vi "Actor Core.vi"(8 "error in":errorcluster, 11 "BuildServer in":refnum<class "BuildServer.lvclass">) -> (0 "error out":errorcluster, 3 "Actor out":refnum<class "Actor.lvclass">)   [LabVIEW 2017, in "BuildServer.lvlib" / "BuildServer.lvclass"]
doc: "(<B>Filename</B>: Actor Framework.lvlib:Actor.lvclass:Actor Core.vi)\n\nReceives messages to the actor, reacts to them, and initiates any error handling that may shut the actor down.\n\nDescendant classes may override this VI to append parallel tasks for the actor to complete while it handles messages. Overrides use the Call Parent Method node."
uses:
  BuildServer.lvclass
  <vilib>/ActorFramework/Actor/Actor.lvclass
  BuildServer Messages/Add LVProject Msg/Add LVProject Msg.lvclass
  BuildServer Messages/Update Project Organization Msg/Update Project Organization Msg.lvclass
  BuildServer Messages/Remove LVProject Msg/Remove LVProject Msg.lvclass
  BuildServer Messages/Add Tasks Msg/Add Tasks Msg.lvclass
  BuildServer Messages/Remove Tasks Msg/Remove Tasks Msg.lvclass
  BuildServer Messages/Sort TaskView Msg/Sort TaskView Msg.lvclass
  BuildServer Messages/Launch Task Settings Msg/Launch Task Settings Msg.lvclass
  <vilib>/ActorFramework/Stop Msg/Stop Msg.lvclass
  BuildServer Messages/Send Tasks To Workers Msg/Send Tasks To Workers Msg.lvclass
  BuildServer Messages/Start Tasks Msg/Start Tasks Msg.lvclass
  BuildServer Messages/Cancel Tasks Msg/Cancel Tasks Msg.lvclass
  BuildServer Messages/Stop Worker Msg/Stop Worker Msg.lvclass
  BuildServer Messages/Worker List Menu Selection Msg/Worker List Menu Selection Msg.lvclass
  <vilib>/Utility/sysdir.llb/System Directory Type.ctl
  BuildServer Messages/Task Update Message Msg/Task Update Message Msg.lvclass
  WebSocket Server/Actors/Actor wHelper/Actor wHelper/Actor wHelper.lvclass
  Volumes/Data/Users/benji667/Git/BuildFarm/WebSocket Server/Actors/Actor wHelper/Actor wHelper/Actor wHelper.lvclass
  Volumes/Data/Users/benji667/Git/BuildFarm/WebSocket Server/Actors/Actor wHelper/Actor wLauncher/Actor wLauncher.lvclass
  Volumes/Data/Users/benji667/Git/BuildFarm/WebSocket Server/Actors/Actor wHelper/Actor wUI/Actor wUI.lvclass
  Applications/National Instruments/LabVIEW 2017 64-bit/vi.lib/ActorFramework/Actor/Actor.lvclass
  ProjectOrganization.ctl
panel:
  in  "tasksSend":bool
  in  "projectsDelete":bool
  in  "tasksAdd":bool
  in  "projectsOpen":bool
  in  "tasksRemove":bool
  in  "workerKill":bool
  in  "taskSettings":bool
  in  "taskCancel":bool
  in  "taskStart":bool
  in  "projectOrganization":T1
  in  "ProjectsView":string[](tree)
  in  "TasksView":i32[](listbox)
  out "Status":string
  out "#proc":i32 caption="# of logical processors"
  out "WorkerList":string[][](array[string])
  # "LabVIEW Projects"
  # "Tasks"
  # "Status"
  # "Workers"
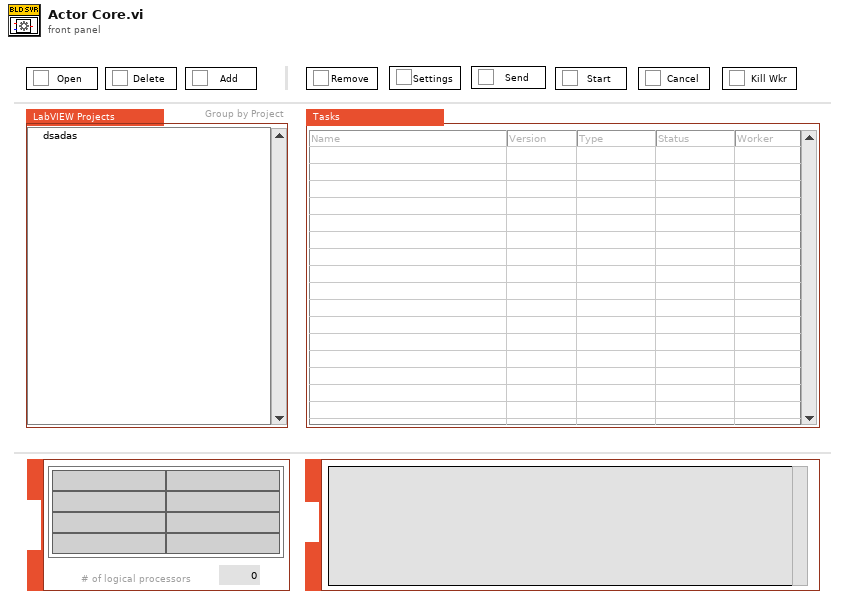
[diagram p1: front panel]
types:
  T1 = typedef "BuildServer.lvlib/BuildServer.lvclass/ProjectOrganization.ctl" = enum16{"Group by Project", "Group by Target", "Group by Type", "Group by Name"}
  T2 = cluster{"Properties:StopHelperLoop Reg Ref":refnum<event-registration>, "Properties:Msg Update Event":refnum<event-registration>, "Properties:New Worker Event":refnum<event-registration>}
  T3 = typedef "System Directory Type.ctl" = i32
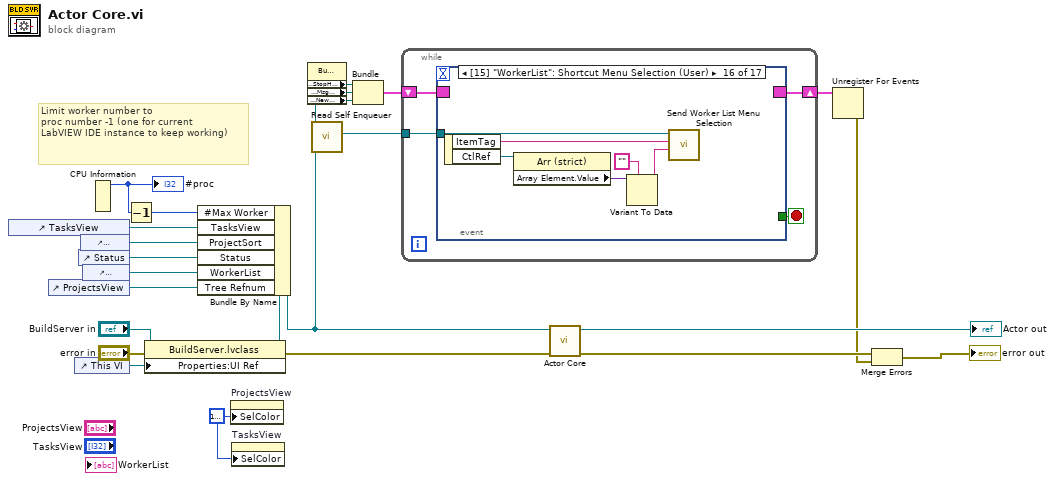
[diagram p0: block diagram]
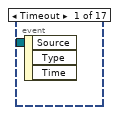
[diagram p2: hidden frame]
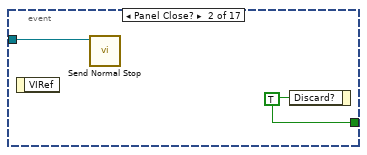
[diagram p3: hidden frame]
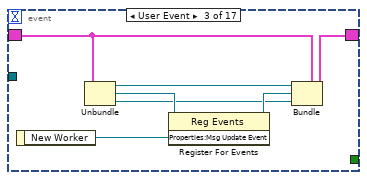
[diagram p4: hidden frame]
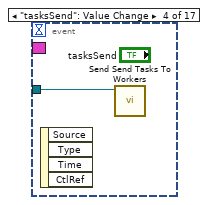
[diagram p5: hidden frame]
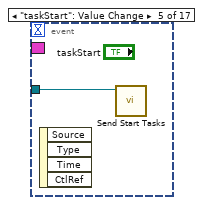
[diagram p6: hidden frame]
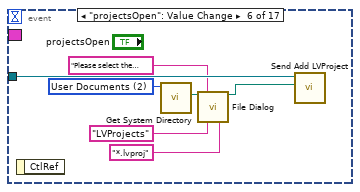
[diagram p7: hidden frame]
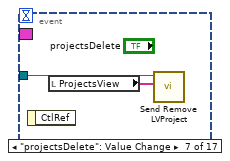
[diagram p8: hidden frame]
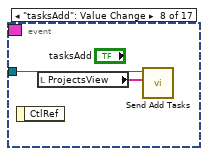
[diagram p9: hidden frame]
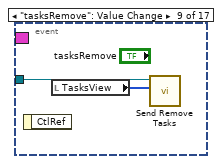
[diagram p10: hidden frame]
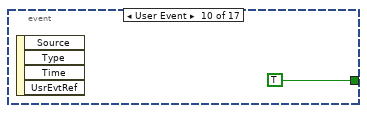
[diagram p11: hidden frame]
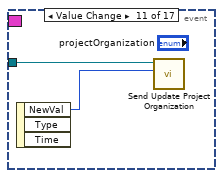
[diagram p12: hidden frame]
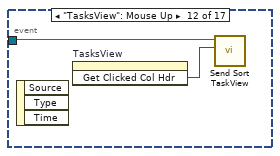
[diagram p13: hidden frame]
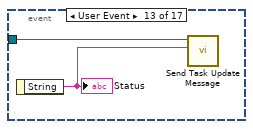
[diagram p14: hidden frame]
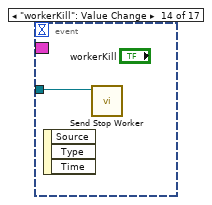
[diagram p15: hidden frame]
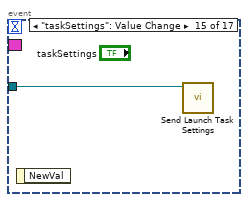
[diagram p16: hidden frame]
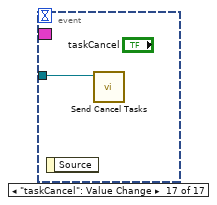
[diagram p17: hidden frame]
diagram:
  w13 = u32 16777224 ("Selection Color")
  # "Limit worker number to\nproc number -1 (one for current\nLabVIEW IDE instance to keep working)"
  n1 = control-ref of="TasksView"() -> (w14:refnum<vi>)
  n2 = control-ref of="ProjectsView"() -> (w19:refnum<vi>)
  n3 = control-ref of="This VI"() -> (w3:refnum<vi>)
  n4 = control-ref of="Status"() -> (w16:refnum<vi>)
  n5 = control-ref of="projectOrganization"() -> (w15:refnum<vi>)
  n6 = control-ref of="WorkerList"() -> (w17:refnum<vi>)
  n7 = CPU Information() -> (4:w10:i32)  [unwired: 3 out]
  "#proc" <- w10
  n8 = Decrement(x=w10) -> (x-1=w9:i32)
  n9 = property class="BuildServer.lvclass"(reference="BuildServer in", error in="error in", "Properties:UI Ref"=w3) -> (reference out=w5:refnum<class "BuildServer.lvclass">, error out=w1:errorcluster)
  n10 = Bundle By Name(cluster=w5, "#Max Worker"=w9, "TasksView"=w14, "ProjectSort"=w15, "Status"=w16, "WorkerList"=w17, "Tree Refnum"=w19) -> (w2:refnum<class "BuildServer.lvclass">)
  n11 = property on="ProjectsView" class="Tree (strict)"("SelColor"=w13) -> ()  [unwired: 2 in, 2 out]
  n12 = property on="TasksView" class="MCListbox (strict)"("SelColor"=w13) -> ()  [unwired: 2 in, 2 out]
  n13 = property class="BuildServer.lvclass"(reference=w2) -> ("Properties:StopHelperLoop Reg Ref"=w21:refnum<event-registration>, "Properties:Msg Update Event"=w8:refnum<event-registration>, "Properties:New Worker Event"=w6:refnum<event-registration>)  [unwired: 1 in, 2 out]
  n14 = call <vilib>:"Read Self Enqueuer.vi"("Actor"=w2) -> ("Self Enqueuer"=w18:refnum<class "Message Enqueuer.lvclass">)  [unwired: 10 in]
  n15 = Bundle("Properties:StopHelperLoop Reg Ref"=w21, "Properties:Msg Update Event"=w8, "Properties:New Worker Event"=w6) -> (w20:T2)  [unwired: 1 in]
  n16 = while {
    tunnel: w18 -> [w26]
    shift-right: [w25] -> w7
    shift-left: w20 -> [w27]
    stop <- w28 stop-if-true
    n17 = event shown="[15] \"WorkerList\": Shortcut Menu Selection (User)" {
      selector: w27 -> [_ _ w37 _ _ _ _ _ _ _ _ _ _ _ _ _ _]
      dyn-events: [_ _ w35 _ _ _ _ _ _ _ _ _ _ _ _ _ _] -> w25
      timeout: _ -> [_ _ _ _ _ _ _ _ _ _ _ _ _ _ _ _ _]
      tunnel: [_ w30 _ _ _ _ _ _ _ TRUE ("Discard?") _ _ _ _ _ _ _] -> w28
      tunnel: w26 -> [_ w29 _ w38 w39 w46 w48 w50 w52 _ w55 w57 w59 w60 w61 w64 w68]
      event Timeout {
        n18 = event-data() -> ()  [unwired: 1 in, 3 out]
      }
      event Panel Close? {
        w30 = TRUE ("Discard?")
        n19 = event-data() -> ()  [unwired: 1 in, 1 out]
        n20 = call <vilib>:"Send Normal Stop.vi"("Message Enqueuer"=w29) -> ()  [unwired: 10 in, 1 out]
        n21 = event-data("Discard?"=w30) -> ()  [unwired: 1 in, 1 out]
      }
      event User Event {
        n22 = event-data() -> ("New Worker"=w31:refnum<user-event>)  [unwired: 1 in]
        n23 = Unbundle(w37) -> ("Properties:StopHelperLoop Reg Ref"=w34:refnum<event-registration>, "Properties:Msg Update Event"=w36:refnum<event-registration>, "Properties:New Worker Event"=w32:refnum<event-registration>)
        n24 = register-events(reference=w36, w31) -> (reference out=w33:refnum<event-registration>)  [unwired: 1 in, 1 out]
        n25 = Bundle(cluster=w37, "Properties:StopHelperLoop Reg Ref"=w34, "Properties:Msg Update Event"=w33, "Properties:New Worker Event"=w32) -> (w35:T2)
      }
      event "tasksSend": Value Change {
        n26 = event-data() -> ()  [unwired: 1 in, 4 out]
        n27 = call "Send Send Tasks To Workers.vi"("Message Enqueuer"=w38) -> ()  [unwired: 9 in, 2 out]
      }
      event "taskStart": Value Change {
        n28 = event-data() -> ()  [unwired: 1 in, 4 out]
        n29 = call "Send Start Tasks.vi"("Message Enqueuer"=w39) -> ()  [unwired: 9 in, 2 out]
      }
      event "projectsOpen": Value Change {
        w44 = T3 2 items=["User Home"=0, "User Desktop"=1, "User Documents"=2, "User Application Data"=3, "User Preferences"=4, "User Temporary"=5, "Public Documents"=6, "Public Application Data"=7, "Public Preferences"=8, "Public Cache"=13, "System Core Libraries"=9, "System Installed Libraries"=10, "Application Files"=11, "Boot Volume Root"=12] ("system directory type")
        n30 = event-data() -> ()  [unwired: 1 in, 1 out]
        n31 = call <vilib>:"Get System Directory.vi"("system directory type"=w44) -> ("system directory"=w45:path)  [unwired: 10 in]
        n32 = call "File Dialog"("start path"=w45, "prompt"="Please select the LabVIEW project you want to load.", "pattern (all files)"="LVProjects", "pattern label"="*.lvproj") -> ("selected path"=w40:path)  [unwired: 8 in, 3 out]
        n33 = call "Send Add LVProject.vi"("Project Path"=w40, "Message Enqueuer in"=w46) -> ()  [unwired: 8 in, 2 out]
      }
      event "projectsDelete": Value Change {
        n34 = event-data() -> ()  [unwired: 1 in, 1 out]
        n35 = local read "ProjectsView"() -> (w47:string[])
        n36 = call "Send Remove LVProject.vi"("User Selections"=w47, "Message Enqueuer in"=w48) -> ()  [unwired: 8 in, 2 out]
      }
      event "tasksAdd": Value Change {
        n37 = event-data() -> ()  [unwired: 1 in, 1 out]
        n38 = local read "ProjectsView"() -> (w49:string[])
        n39 = call "Send Add Tasks.vi"("User Selections"=w49, "Message Enqueuer in"=w50) -> ()  [unwired: 8 in, 2 out]
      }
      event "tasksRemove": Value Change {
        n40 = event-data() -> ()  [unwired: 1 in, 1 out]
        n41 = local read "TasksView"() -> (w51:i32[])
        n42 = call "Send Remove Tasks.vi"("User Selections"=w51, "Message Enqueuer"=w52) -> ()  [unwired: 8 in, 2 out]
      }
      event User Event {
        n43 = event-data() -> ()  [unwired: 1 in, 4 out]
      }
      event Value Change {
        n44 = event-data() -> ("NewVal"=w54:T1)  [unwired: 1 in, 2 out]
        n45 = call "Send Update Project Organization.vi"("ProjectOrganization"=w54, "Message Enqueuer in"=w55) -> ()  [unwired: 8 in, 2 out]
      }
      event "TasksView": Mouse Up {
        n46 = event-data() -> ()  [unwired: 1 in, 3 out]
        n47 = invoke on="TasksView" class="MCListbox (strict)" method="Get Clicked Col Hdr"() -> ("Get Clicked Column Header"=w56:i32)  [unwired: 3 in, 2 out]
        n48 = call "Send Sort TaskView.vi"("Clicked Column"=w56, "Message Enqueuer"=w57) -> ()  [unwired: 8 in, 2 out]
      }
      event User Event {
        n49 = event-data() -> ("String"=w58:string)  [unwired: 1 in]
        "Status" <- w58
        n50 = call "Send Task Update Message.vi"("Task Update Message"=w58, "Message Enqueuer"=w59) -> ()  [unwired: 8 in, 2 out]
      }
      event "workerKill": Value Change {
        n51 = event-data() -> ()  [unwired: 1 in, 3 out]
        n52 = call "Send Stop Worker.vi"("Message Enqueuer"=w60) -> ()  [unwired: 9 in, 2 out]
      }
      event "taskSettings": Value Change {
        n53 = event-data() -> ()  [unwired: 1 in, 1 out]
        n54 = call "Send Launch Task Settings.vi"("Message Enqueuer"=w61) -> ()  [unwired: 9 in, 2 out]
      }
      event "WorkerList": Shortcut Menu Selection (User) {
        n55 = event-data() -> ("ItemTag"=w63:string, "CtlRef"=w67:refnum<vi>)  [unwired: 1 in]
        n56 = property class="Arr (strict)"(reference=w67) -> ("Array Element.Value"=w66:variant)  [unwired: 1 in, 2 out]
        n57 = Variant To Data(type="", Variant=w66) -> (data=w62:string)  [unwired: 1 in, 1 out]
        n58 = call "Send Worker List Menu Selection.vi"("Worker Name"=w62, "Menu Item Tag"=w63, "Message Enqueuer"=w64) -> ()  [unwired: 7 in, 2 out]
      }
      event "taskCancel": Value Change {
        n59 = event-data() -> ()  [unwired: 1 in, 1 out]
        n60 = call "Send Cancel Tasks.vi"("Message Enqueuer"=w68) -> ()  [unwired: 9 in, 2 out]
      }
    }
  }
  n61 = call-parent "Actor Core.vi"("error in"=w1, "Actor in"=w2) -> ("error out"=w24:errorcluster, "Actor out"=→"Actor out":refnum<class "Actor.lvclass">)  [unwired: 8 in]
  n62 = Unregister For Events(event registration refnum=w7) -> (error out=w11:errorcluster)  [unwired: 1 in]
  n63 = Merge Errors(w24, w11) -> (→"error out":errorcluster)
